vi "ParseControlDescription.vi"(5 "label":string, 9 "Control description":string) -> (1 "description":string, 2 "flags":string[](array[string]), 3 "position":i32)   [LabVIEW 2014, in "Raspberry Pi Compatible Compiler for LabVIEW.lvlib" / "PyConvBD.lvclass"]
uses:
  PyConvBD.lvclass
  <vilib>/regexp/Match Regular Expression.xnode
  Parsing/Python Functions.lvlib
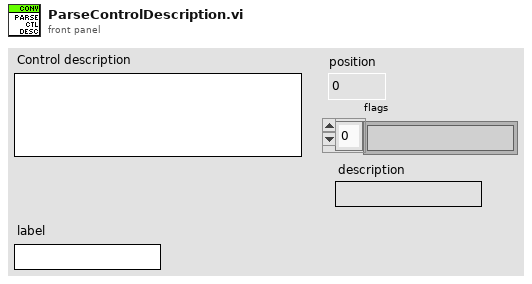
[diagram p1: front panel]
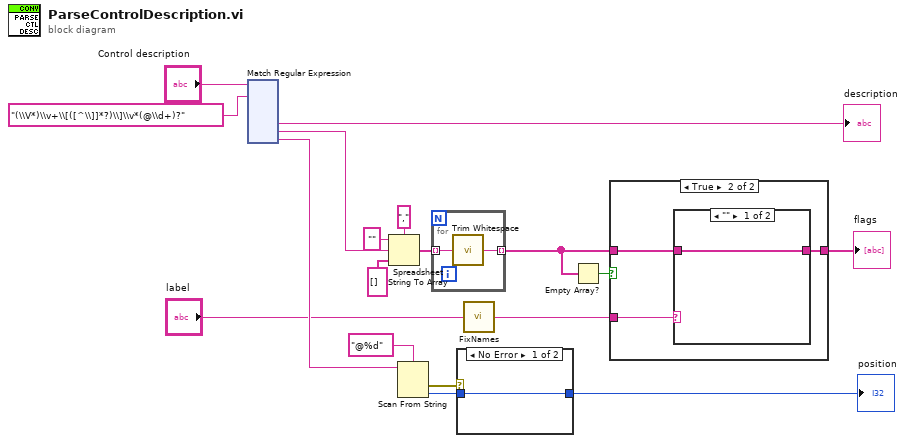
[diagram p0: block diagram]
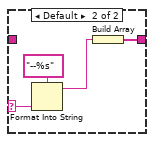
[diagram p3: hidden frame]
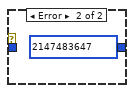
[diagram p4: hidden frame]
diagram:
  n1 = xnode "Match Regular Expression"("input string"="Control description", "regular expression"="(\\V*)\\v+\\[([^\\]]*?)\\]\\v*(@\\d+)?") -> ("submatch 1"=→"description":string, "submatch 2"=w16:string, "submatch 3"=w11:string)  [unwired: 4 in, 5 out]
  n2 = Spreadsheet String To Array(delimiter (Tab)=",", format string="", spreadsheet string=w16, array type (2D Dbl)=string[] []) -> (array=w12:string[])
  n3 = Scan From String(format string="@%d", input string=w11) -> (error out=w9:errorcluster, output 1=w8:i32)  [unwired: 3 in, 2 out]
  n4 = for {
    tunnel: w12 -> [w20] mode=indexing
    tunnel: [w19] -> w1 mode=indexing
    n5 = call <vilib>:"Trim Whitespace.vi"("string"=w20) -> ("trimmed string"=w19:string)  [unwired: 1 in]
  }
  n6 = case shown="No Error" w9 {
    tunnel: w8 -> [w21 _]
    tunnel: [w21 2147483647] -> w4
    frame No Error {
    }
    frame Error {
    }
  }
  "position" <- w4
  n7 = call "FixNames.vi"("name"="label") -> ("python name"=w6:string)
  n8 = Empty Array?(array=w1) -> (empty?=w2:bool)
  n9 = case shown="True" w2 {
    tunnel: w1 -> [w23 w26]
    tunnel: w6 -> [_ w25]
    tunnel: [w23 w24] -> w3
    frame False {
    }
    frame True {
      n10 = case shown="\"\"" w25 {
        selector: w25 -> [_ w30]
        tunnel: w26 -> [w27 _]
        tunnel: [w27 w31] -> w24
        frame "" {
        }
        frame Default {
          n11 = Format Into String(format string="--%s", w30) -> (resulting string=w29:string)  [unwired: 2 in, 1 out]
          n12 = Build Array(w29) -> (w31:string[])
        }
      }
    }
  }
  "flags" <- w3
